vi "Chirp directives Generated.vi"(5 "Real In":cluster{"element":fxp<+/-,64,32>, "valid?":bool}, 7 "Imaginary In":cluster{"element":fxp<+/-,64,32>, "valid?":bool}, 9 "input valid":bool=TRUE, 12 "Chirp/Fft Pair 1 - Chirp Rate":fxp<+/-,64,32>) -> (6 "Chirped Real Out":cluster{"element":fxp<+/-,64,32>, "valid?":bool}, 8 "Chirped Imaginary Out":cluster{"element":fxp<+/-,64,32>, "valid?":bool}, 14 "feedback signals":T1)   [LabVIEW 2012]
doc: "This VI is created by the LabVIEW 2012 FPGA IP Builder.\n\nProject: seti_labview.lvproj\nTarget: FPGA Target (PXI-7953R)/IP Builder\nBuild Specification: Chirp directives\nDirectives Item: Chirp directives\nTop-Level VI: C:\\work\\seti_fpga\\LabVIEW\\Tester\\SETI_LV_FPGA\\Chirp.vi\n\nEstimated Device Utilization\n-------------------------------------\nSlice Registers: 5.7% (2933 out of 51840)\nSlice LUTs: 6.4% (3330 out of 51840)\nDSP48s: 50.0% (24 out of 48)\nBlock RAMs: 3.6% (7 out of 192)\n\nEstimated Performance\n-------------------------------------\nClock rate (MHz): 250.63\nInitiation interval (cycles): 986\nPipeline type: Not pipelined\nMinimum latency: 985\nMaximum latency: 985"
uses:
  <vilib>/rvi/IPIntegrationNode/IPINode_Utilities/niFpgaIPINodeSimCore.vi
  <vilib>/rvi/IPIntegrationNode/IPINode_Xnode/niFpgaIPINode.xnode
  Chirp directives Generated Support/IPBlockSimFiles/mF9414AA7_topH_7B4C49CEC4DA4D169525EFFCDC5DA652.dll
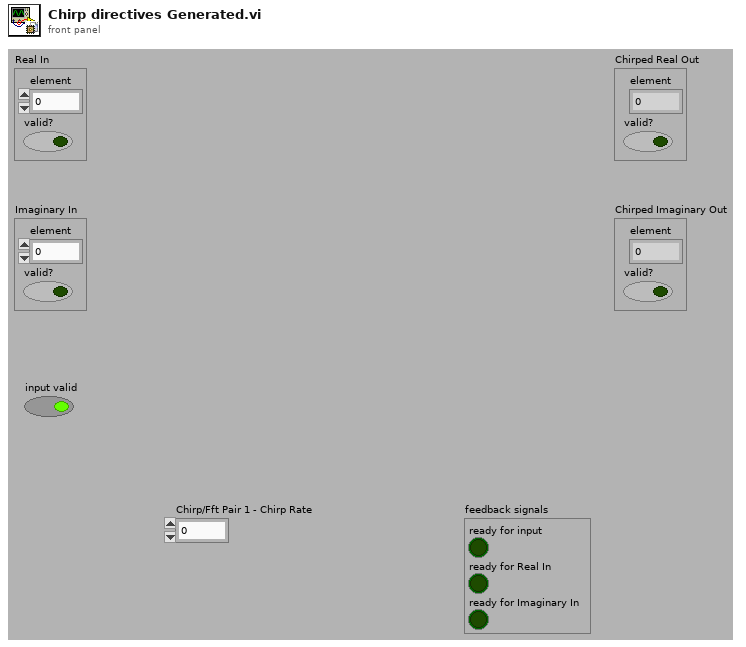
[diagram p1: front panel]
types:
  T1 = cluster{"ready for input":bool, "ready for Real In":bool, "ready for Imaginary In":bool}
  T2 = cluster{"p_Chirped_Real_Out_2_V_din":fxp<+/-,64,32>, "p_Chirped_Real_Out_2_vld":bool}
  T3 = cluster{"p_Chirped_Imaginary_Out_1_V_din":fxp<+/-,64,32>, "p_Chirped_Imaginary_Out_1_vld":bool}
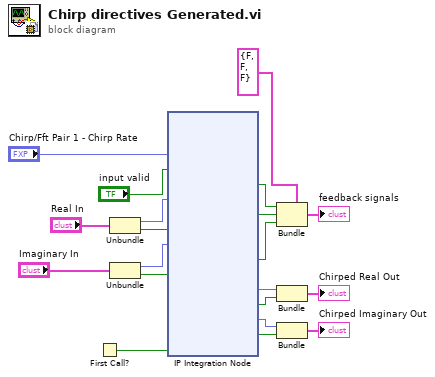
[diagram p0: block diagram]
diagram:
  n1 = First Call?() -> (First Call?: T/F=w20:bool)
  n2 = Unbundle("Real In") -> ("element"=w13:fxp<+/-,64,32>, "valid?"=w12:bool)
  n3 = Unbundle("Imaginary In") -> ("element"=w9:fxp<+/-,64,32>, "valid?"=w8:bool)
  n4 = xnode "IP Integration Node"("p_Chirp_slash_Fft_Pair_1_dash_Chirp_Rate_6_V"="Chirp/Fft Pair 1 - Chirp Rate", "input_valid"="input valid", "p_Real_In_10_V_dout"=w13, "p_Real_In_10_vld"=w12, "p_Imaginary_In_9_V_dout"=w9, "p_Imaginary_In_9_vld"=w8, "first_call"=w20) -> ("ready_for_input"=w17:bool, "ready_for_p_Real_In_10"=w11:bool, "ready_for_p_Imaginary_In_9"=w7:bool, "p_Chirped_Real_Out_2_V_din"=w5:fxp<+/-,64,32>, "p_Chirped_Real_Out_2_vld"=w4:bool, "p_Chirped_Imaginary_Out_1_V_din"=w2:fxp<+/-,64,32>, "p_Chirped_Imaginary_Out_1_vld"=w1:bool)  [unwired: 2 in]
  n5 = Bundle ("Bundle_feedback")(cluster=T1 {"ready for input"=FALSE, "ready for Real In"=FALSE, "ready for Imaginary In"=FALSE}, "ready for input"=w17, "ready for Real In"=w11, "ready for Imaginary In"=w7) -> (→"feedback signals":T1)
  n6 = Bundle("p_Chirped_Real_Out_2_V_din"=w5, "p_Chirped_Real_Out_2_vld"=w4) -> (→"Chirped Real Out":T2)  [unwired: 1 in]
  n7 = Bundle("p_Chirped_Imaginary_Out_1_V_din"=w2, "p_Chirped_Imaginary_Out_1_vld"=w1) -> (→"Chirped Imaginary Out":T3)  [unwired: 1 in]
